vi "GetIdentity.vi"(8 "error in (no error)":errorcluster, 11 "SMO in":refnum<class "SMO.lvclass">) -> (0 "error out":errorcluster, 1 "GUID":string, 2 "Name":string, 3 "SMO out":refnum<class "SMO.lvclass">)   [LabVIEW 2013, in "SMO.lvclass"]
uses:
  SMO.lvclass
  Support/Attribute.Identity/Attribute.Identity.lvclass
  Support/Attribute.Identity/Attribute.Identity.lvclass/Attribute.Identity.ctl
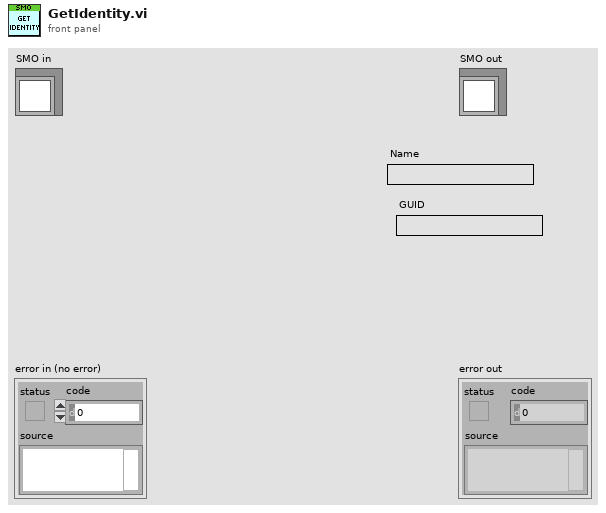
[diagram p1: front panel]
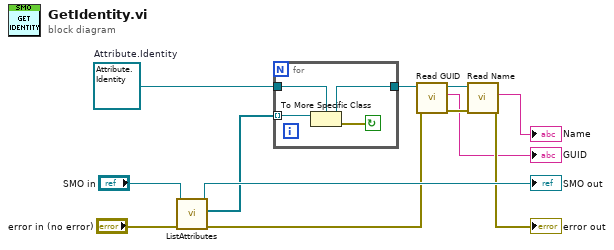
[diagram p0: block diagram]
diagram:
  w8 = refnum<class "Attribute.Identity.lvclass"> refnum  # Attribute.Identity
  n1 = call "ListAttributes.vi"("error in (no error)"="error in (no error)", "SMO in"="SMO in") -> ("error out"=w5:errorcluster, "[Attributes]"=w9:refnum<class "Attribute.lvclass">[], "SMO out"=→"SMO out":refnum<class "SMO.lvclass">)  [unwired: 7 in]
  n2 = for {
    tunnel: w9 -> [w16] mode=indexing
    tunnel: w8 -> [w15]
    tunnel: [w13] -> w7
    stop <- w14 continue-if-true
    n3 = To More Specific Class(target class=w15, reference=w16) -> (specific class reference=w13:refnum<class "Attribute.Identity.lvclass">, error out=w14:errorcluster)  [unwired: 1 in]
  }
  n4 = call "Read GUID.vi"("error in (no error)"=w5, "Attribute.Identity in"=w7) -> ("error out"=w4:errorcluster, "GUID"=→"GUID":string, "Attribute.Identity out"=w6:refnum<class "Attribute.Identity.lvclass">)  [unwired: 7 in]
  n5 = call "Read Name.vi"("error in (no error)"=w4, "Attribute.Identity in"=w6) -> ("error out"=→"error out":errorcluster, "Name"=→"Name":string)  [unwired: 7 in, 1 out]
